vi "Configure Measurement Name.vi"(8 "error in (no error)":errorcluster, 9 "Measurement Name (Q-factor(rc))":string="Q-factor(rc)", 10 "Measurement Position (1: Position 1)":i32(ring)=1 items=["Position 1"=1, "Position 2"=2, "Position 3"=3, "Position 4"=4, "Position 5"=5, "Position 6"=6, "Position 7"=7, "Position 8"=8, "Position 9"=9, "Position 10"=10], 11 "VISA resource name":refnum<visa-resource-name>) -> (0 "error out":errorcluster, 3 "VISA resource name out":refnum<visa-resource-name>)   [LabVIEW 2013, in "Agilent 90000 Series.lvlib"]
doc: "Sets the name of the specified measurement to whatever string is given to <name>. This lets you give specific names to measurements displayed on the oscilloscope's screen.\n\n<b>Note:</b> This VI is new in firmware version 4.50."
uses:
  Agilent 90000 Series.lvlib
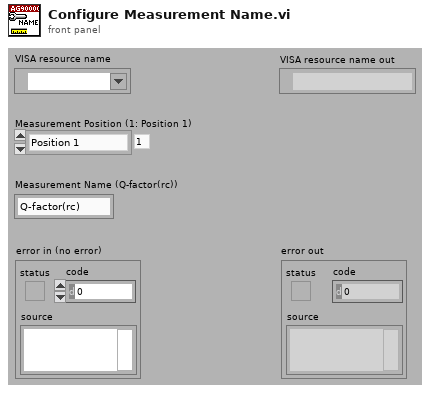
[diagram p1: front panel]
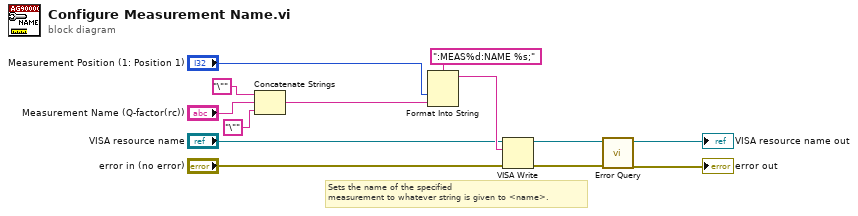
[diagram p0: block diagram]
diagram:
  # "Sets the name of the specified\nmeasurement to whatever string is given to <name>."
  n1 = Concatenate Strings("\"" ("string"), "Measurement Name (Q-factor(rc))", "\"" ("string")) -> (w2:string)
  n2 = Format Into String(format string=":MEAS%d:NAME %s;", "Measurement Position (1: Position 1)", w2) -> (resulting string=w12:string)  [unwired: 2 in, 1 out]
  n3 = VISA Write(VISA resource name="VISA resource name", write buffer=w12, error in (no error)="error in (no error)") -> (VISA resource name out=w9:refnum<visa-resource-name>, error out=w8:errorcluster)  [unwired: 1 out]
  n4 = call "Error Query.vi"("error in (no error)"=w8, "VISA resource name"=w9) -> ("error out"=→"error out":errorcluster, "VISA resource name out"=→"VISA resource name out":refnum<visa-resource-name>)  [unwired: 6 in, 2 out]
